vi "led_matr_v2.vi"() -> ()   [LabVIEW 2009]
panel:
  out "Coloana selectata":bool[](array[boolean])=[FALSE, TRUE, FALSE, FALSE, FALSE, TRUE, FALSE]
  in  "Array 3":bool[][](array[boolean])=[[FALSE, TRUE, TRUE, TRUE, FALSE], [TRUE, FALSE, FALSE, FALSE, TRUE], [FALSE, FALSE, FALSE, FALSE, TRUE], [FALSE, FALSE, TRUE, TRUE, FALSE], [FALSE, FALSE, FALSE, FALSE, TRUE], [TRUE, FALSE, FALSE, FALSE, TRUE], [FALSE, TRUE, TRUE, TRUE, FALSE]]
  out "Coloana":u8(slide) scale=0.0..4.0
  in  "Iesire":bool
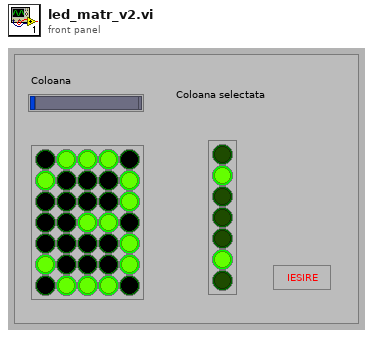
[diagram p1: front panel]
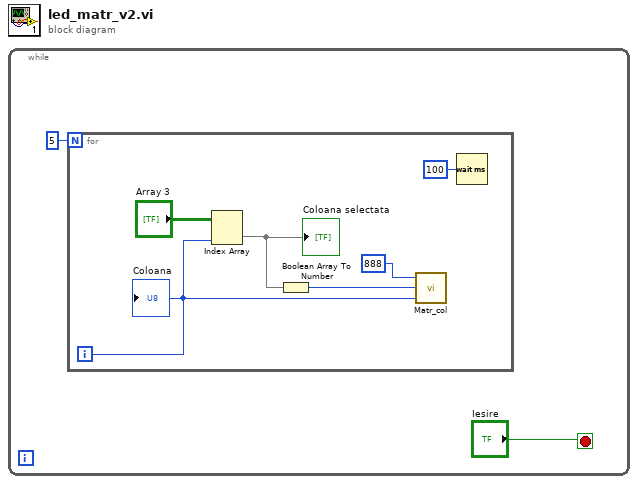
[diagram p0: block diagram]
diagram:
  n1 = while {
    stop <- "Iesire" stop-if-true
    n2 = for {
      N: 5 -> [_]
      i -> [w4]
      n3 = Index Array(array="Array 3", index (col)=w4) -> (element=w6:bool[])  [unwired: 1 in]
      "Coloana selectata" <- w6
      n4 = Boolean Array To Number(Boolean array=w6) -> (number=w5:u32)
      n5 = call "Matr_col.vi"("Coloana"=w4, "Date"=w5, "Adresa"=u32 888 ("milliseconds to wait")) -> ()  [unwired: 2 out]
      n6 = Wait (ms)(milliseconds to wait=u32 100) -> ()  [unwired: 1 out]
      "Coloana" <- w4
    }
  }
